vi "Stop Core.vi"(10 "final error code":i32, 11 "Actor wHelper in":refnum<class "Actor wHelper.lvclass">) -> (3 "Actor wHelper out":refnum<class "Actor wHelper.lvclass">)   [LabVIEW 2017, in "Framework.lvlib" / "Actor wHelper.lvclass"]
doc: "(<B>Filename</B>: Actor Framework.lvlib:Actor.lvclass:Stop Core.vi)\n\nDefines what the actor does before it stops. Use the <B>final error code</B> input to determine whether the actor shut down in response to an error.\n\nBy default, this method does nothing. A descendant class may override it to define behavior, such as shutting down any processes the actor initiated in its override of the Actor Core method."
uses:
  Actor wHelper.lvclass
  Actor wHelper.lvclass/Actor wHelper.ctl
  Actor wLauncher/Actor wLauncher.lvclass
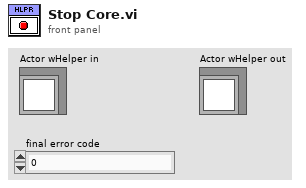
[diagram p1: front panel]
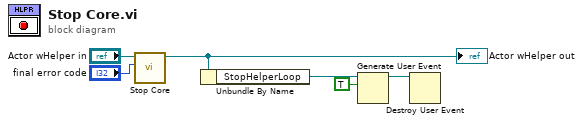
[diagram p0: block diagram]
diagram:
  n1 = call-parent "Stop Core.vi"("final error code"="final error code", "Actor wUI in"="Actor wHelper in") -> ("Actor wUI out"=w2:refnum<class "Actor wHelper.lvclass">)  [unwired: 9 in]
  "Actor wHelper out" <- w2
  n2 = Unbundle By Name(w2) -> ("StopHelperLoop"=w1:refnum<user-event>)
  n3 = Generate User Event(user event=w1, event data cluster=TRUE ("event data")) -> (user event out=w3:refnum<user-event>)  [unwired: 2 in, 1 out]
  n4 = Destroy User Event(user event=w3) -> ()  [unwired: 1 in, 1 out]
